vi "SMS data FGV.vi"(1 "Action":T2, 4 "Power supply data in":T1) -> (0 "Power supply data out":T1)   [LabVIEW 2017, in "Magnet module.lvlib"]
uses:
  ctl/FGV action.ctl
  Magnet module.lvlib
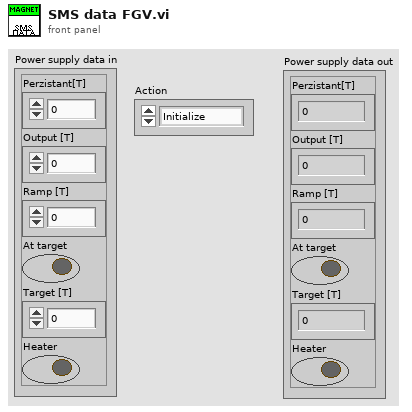
[diagram p1: front panel]
types:
  T1 = cluster{"Perzistant[T]":dbl, "Output [T]":dbl, "Ramp [T]":dbl, "At target":bool, "Target [T]":dbl, "Heater":bool}
  T2 = typedef "Magnet module.lvlib/FGV action.ctl" = enum16{"Initialize", "Update", "Read", "Action"}
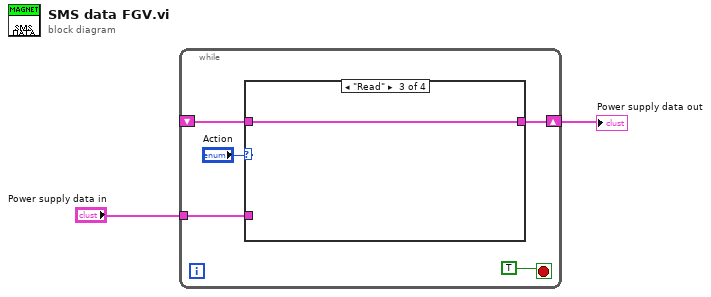
[diagram p0: block diagram]
diagram:
  n1 = while {
    shift-right: [w5] -> w2
    shift-left: _ -> [w6]
    tunnel: "Power supply data in" -> [w4]
    stop <- TRUE stop-if-true
    n2 = case shown="\"Read\"" "Action" {
      tunnel: [w8 w9 w10 w11] -> w5
      tunnel: w6 -> [_ _ w10 w11]
      tunnel: w4 -> [w8 w9 _ _]
      frame "Initialize", Default {
      }
      frame "Update" {
      }
      frame "Read" {
      }
      frame "Action" {
      }
    }
  }
  "Power supply data out" <- w2
